vi "Complex Hessenberg Decomposition.vi"(9 "index high":i32=-1, 10 "index low":i32=-1, 11 "Input Matrix":T1) -> (0 "error":i32, 2 "Orthogonal Matrix Q":T1, 3 "Hessenberg Form H":T1)   [LabVIEW 2017, in "NI_AALPro.lvlib"]
doc: "Performs the Hessenberg decomposition of <B>Input Matrix</B>. Wire data to the <B>Input Matrix</B> input to determine the polymorphic instance to use or manually select the instance."
uses:
  NI_AALPro.lvlib
  ComplexMatrix.ctl
  <resource>/lvanlys.dll
  NI_Matrix.lvlib
panel:
  # "Hessenberg Decomposition"
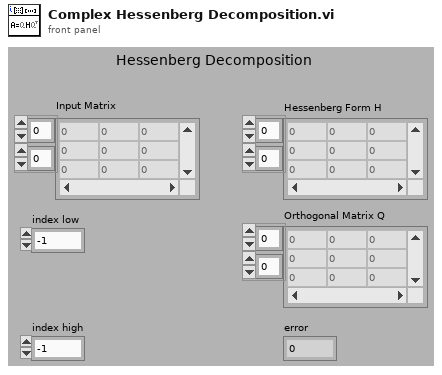
[diagram p1: front panel]
types:
  T1 = typedef "NI_Matrix.lvlib/ComplexMatrix.ctl" = cdb[][]
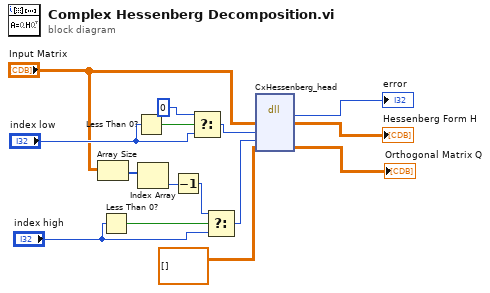
[diagram p0: block diagram]
diagram:
  n1 = Array Size(array="Input Matrix") -> (size(s)=w5:i32[])
  n2 = Less Than 0?(x="index high") -> (x < 0?=w7:bool)
  n3 = Less Than 0?(x="index low") -> (x < 0?=w11:bool)
  n4 = Index Array(array=w5) -> (element=w2:i32)  [unwired: 1 in]
  n5 = Decrement(x=w2) -> (x-1=w1:i32)
  n6 = Select(t=0, s=w11, f="index low") -> (s? t:f=w9:i32)
  n7 = Select(t=w1, s=w7, f="index high") -> (s? t:f=w3:i32)
  n8 = dll-call lib="C:/Program Files (x86)/National Instruments/LabVIEW 2017/resource/lvanlys.*" fn="CxHessenberg_head"("Input Matrix"="Input Matrix", "ilo"=w9, "ihi"=w3, "output param"=cdb[][] []) -> (→"error":i32, "Input Matrix"=→"Hessenberg Form H":T1, "output param"=→"Orthogonal Matrix Q":cdb[][])  [unwired: 5 in, 2 out]
